vi "testNestedEmptyElementAffectingSyblings(Case7440).vi"(8 "error in (no error)":errorcluster, 11 "reference in":refnum<class "EasyXML_XML_Subset_Built_Tests.lvclass">) -> (0 "error out":errorcluster, 3 "reference in":refnum<class "EasyXML_XML_Subset_Built_Tests.lvclass">)   [LabVIEW 2013, in "EasyXML_XML_Subset_Built_Tests.lvclass"]
uses:
  EasyXML_XML_Subset_Built_Tests.lvclass
  EasyXML_XML_Subset_Evaluations/EasyXML_XML_Subset_Evaluations.lvclass
panel:
  in  "a":cluster{"b":cluster{"a":string, "c":string}}={"b"={"a"="", "c"="foo"}}
  out "a":cluster{"b":cluster{"a":string, "c":string}}
  in  "XML String":string="<a>\n  <b>\n    <a/>\n    <c>foo</c>\n  </b>\n</a>"
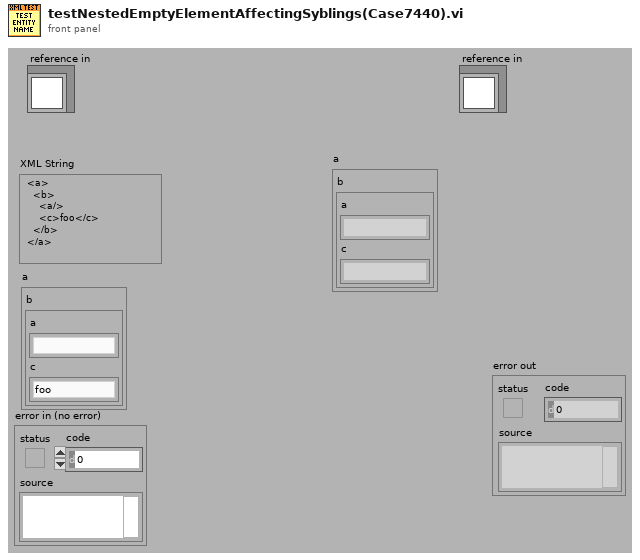
[diagram p1: front panel]
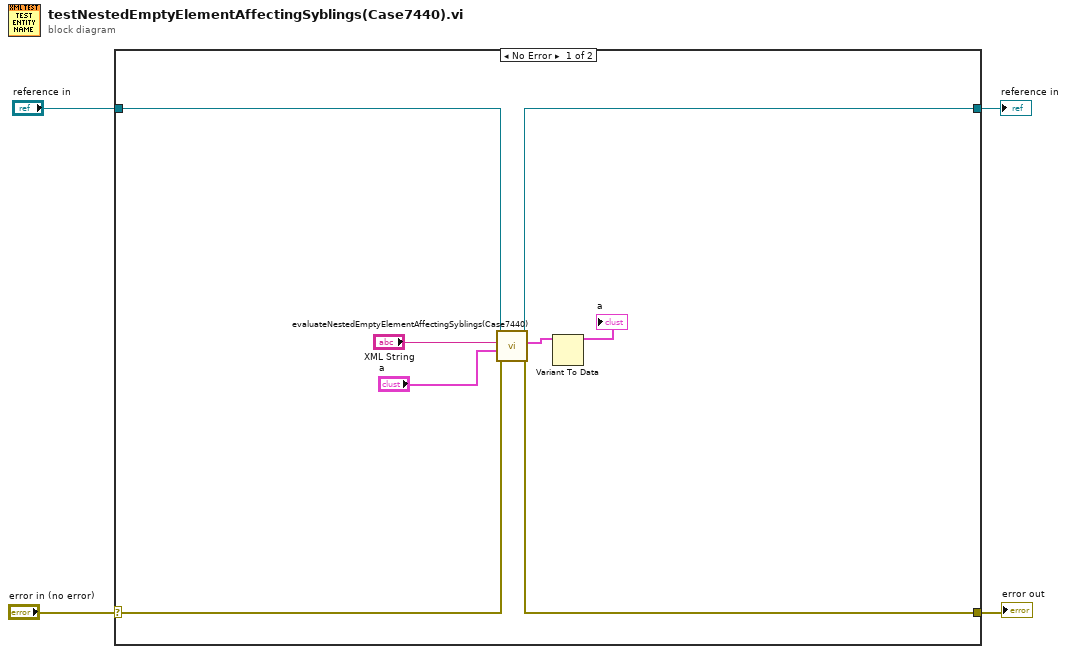
[diagram p0: block diagram]
diagram:
  n1 = case shown="No Error" "error in (no error)" {
    selector: "error in (no error)" -> [w10 w14]
    tunnel: [w6 w14] -> w3
    tunnel: [w11 w13] -> w1
    tunnel: "reference in" -> [w12 w13]
    frame No Error {
      n2 = call "evaluateNestedEmptyElementAffectingSyblings(Case7440).vi"("error in (no error)"=w10, "a"="a", "XML String"="XML String", "reference in"=w12) -> ("error out"=w6:errorcluster, "a"=w8:cluster{"b":cluster{"a":string, "c":string}}, "reference in"=w11:refnum<class "EasyXML_XML_Subset_Built_Tests.lvclass">)  [unwired: 5 in]
      n3 = Variant To Data(Variant=w8) -> (data=→"a":cluster{"b":cluster{"a":string, "c":string}})  [unwired: 2 in, 1 out]
    }
    frame Error {
    }
  }
  "error out" <- w3
  "reference in" <- w1
